vi "Write Data.vi"(5 "Address":T1 format="%02x", 6 "NoStop (F)":bool, 7 "I2C":refnum<class "I2C.lvclass">, 8 "error in (no error)":errorcluster, 10 "Data":string, 11 "Session In":refnum<class "Session.lvclass">) -> (0 "error out":errorcluster, 3 "Session Out":refnum<class "Session.lvclass">)   [LabVIEW 2020, in "CTI.lvlib" / "I2C.lvclass"]
uses:
  I2C.lvclass
  I2C.lvclass/I2C.ctl
  Session/Session.lvclass
  I2C Address.ctl
  CTI.lvlib
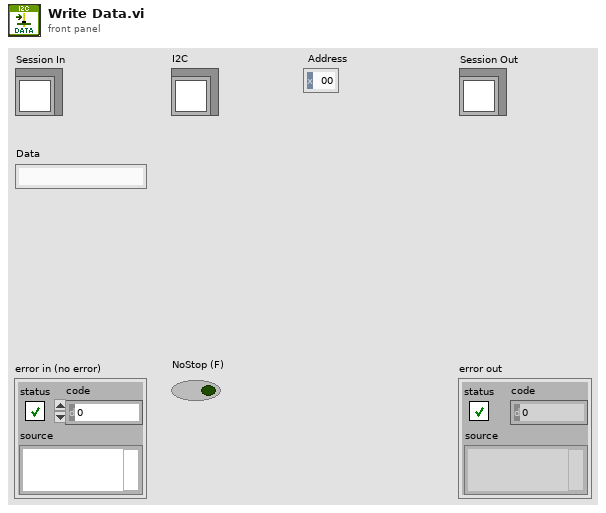
[diagram p1: front panel]
types:
  T1 = typedef "CTI.lvlib/I2C Address.ctl" = u8
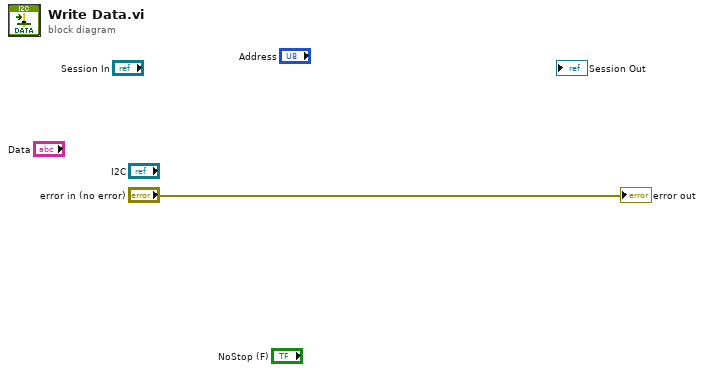
[diagram p0: block diagram]
diagram:
  "error out" <- "error in (no error)"
